vi "未命名 3.vi"() -> ()   [LabVIEW 2017]
panel:
  in  "滑动杆":dbl(slide) scale=0.0..10.0
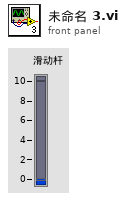
[diagram p1: front panel]
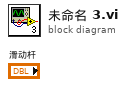
[diagram p0: block diagram]
diagram:
